vi "Library Default Absolute Path.vi"() -> (8 "default absolute path":path)   [LabVIEW 2012]
doc: "Returns the source root when running under the development system or the application directory while built. This absolute path can be used as a default choice for placement of configuration files. To work, this VI must be located two deep under the source root or built into the application."
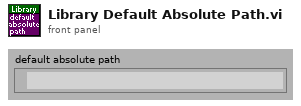
[diagram p1: front panel]
types:
  T1 = enum32{"invalid app kind", "Development System", "Run Time System", "Student Edition", "Embedded LabVIEW", "Evaluation", "Custom"}
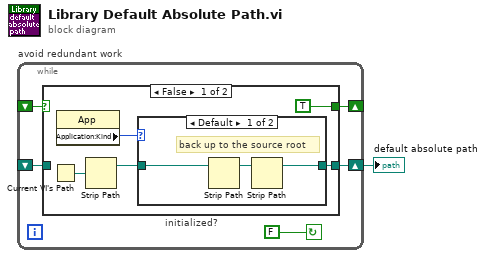
[diagram p0: block diagram]
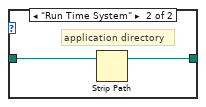
[diagram p2: hidden frame]
diagram:
  n1 = while "avoid redundant work" {
    shift-right: [w2] -> _
    shift-left: _ -> [w3]
    shift-right: [w5] -> w1
    shift-left: _ -> [w4]
    stop <- FALSE continue-if-true
    n2 = case "initialized?" shown="False" w3 {
      selector: w3 -> [_ w17]
      tunnel: [w11 w18] -> w5
      tunnel: w4 -> [_ w18]
      tunnel: [TRUE w17] -> w2
      frame False {
        n3 = Current VI's Path() -> (path=w8:path)
        n4 = property class="App"() -> ("Application:Kind"=w10:T1)  [unwired: 2 in, 2 out]
        n5 = Strip Path(path=w8) -> (stripped path=w7:path)  [unwired: 1 out]
        n6 = case shown="Default" w10 {
          tunnel: [w13 w16] -> w11
          tunnel: w7 -> [w12 w15]
          frame Default {
            # "back up to the source root"
            n7 = Strip Path(path=w12) -> (stripped path=w14:path)  [unwired: 1 out]
            n8 = Strip Path(path=w14) -> (stripped path=w13:path)  [unwired: 1 out]
          }
          frame "Run Time System" {
            # "application directory"
            n9 = Strip Path(path=w15) -> (stripped path=w16:path)  [unwired: 1 out]
          }
        }
      }
      frame True {
      }
    }
  }
  "default absolute path" <- w1
